vi "Get Slew Rates.vi"(0 "reference in":refnum<class "HPS-17000-PowerModule.lvclass">, 11 "Error In":errorcluster) -> (4 "reference out":refnum<class "HPS-17000-PowerModule.lvclass">, 6 "Slew Rates":T1, 15 "Error Out":errorcluster)   [LabVIEW 2023, in "HPS-17000-PowerModule.lvlib" / "HPS-17000-PowerModule.lvclass"]
uses:
  HPS-17000-PowerModule.lvclass
  builds/PowerModuleInterface/PowerModuleInterface.lvlibp/Classes/PowerModule_interface/Slew Rates.ctl
  HPS-17000-PowerModule.lvclass/HPS-17000-PowerModule.ctl
  builds/PowerModuleInterface/PowerModuleInterface.lvlibp/Classes/PowerModule_interface/PowerModuleInterface.lvclass
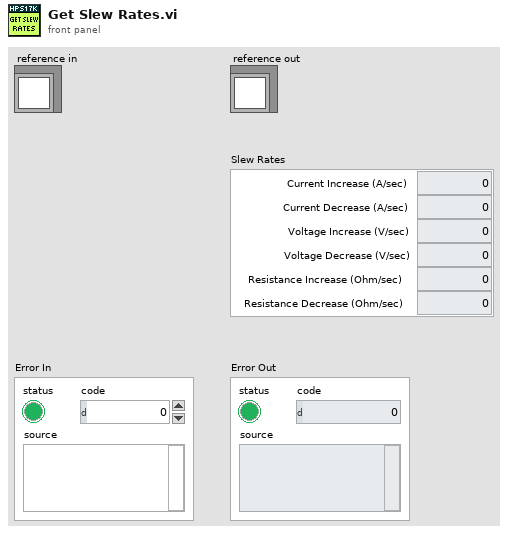
[diagram p1: front panel]
types:
  T1 = typedef "PowerModuleInterface.lvlibp/PowerModuleInterface.lvclass/Slew Rates.ctl" = cluster{"Current Decrease (A/sec)":dbl, "Current Increase (A/sec)":dbl, "Voltage Decrease (V/sec)":dbl, "Voltage Increase (V/sec)":dbl, "Resistance Decrease (Ohm/sec)":dbl, "Resistance Increase (Ohm/sec)":dbl}
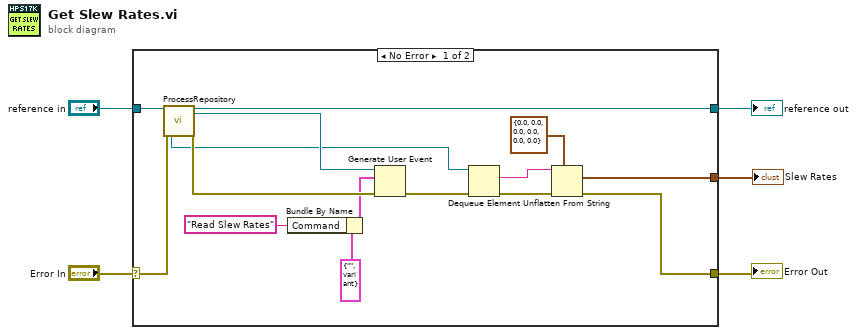
[diagram p0: block diagram]
diagram:
  n1 = case shown="No Error" "Error In" {
    selector: "Error In" -> [w20 w22]
    tunnel: [w9 w22] -> w4
    tunnel: [w18 w21] -> w2
    tunnel: "reference in" -> [w19 w21]
    tunnel: [w6 _] -> w1
    frame No Error {
      n2 = call "ProcessRepository.vi"("reference in"=w19, "Error In"=w20) -> ("QueueFromProcess"=w12:refnum<queue>, "reference out"=w18:refnum<class "HPS-17000-PowerModule.lvclass">, "EventsToProcess"=w17:refnum<user-event>, "Error Out"=w15:errorcluster)  [unwired: 10 in, 4 out]
      n3 = Bundle By Name(cluster=cluster{"Command":string, "Data":variant} {"Command"="", "Data"=variant} ("MessageToProcess"), "Command"="Read Slew Rates") -> (w13:cluster{"Command":string, "Data":variant})
      n4 = Generate User Event(user event=w17, event data cluster=w13, error in=w15) -> (error out=w16:errorcluster)  [unwired: 1 in, 1 out]
      n5 = Dequeue Element(queue=w12, error in (no error)=w16) -> (element=w8:string, error out=w10:errorcluster)  [unwired: 1 in, 2 out]
      n6 = Unflatten From String(type=T1 {"Current Decrease (A/sec)"=0.0, "Current Increase (A/sec)"=0.0, "Voltage Decrease (V/sec)"=0.0, "Voltage Increase (V/sec)"=0.0, "Resistance Decrease (Ohm/sec)"=0.0, "Resistance Increase (Ohm/sec)"=0.0} ("Slew Rates"), binary string=w8, error in (no error)=w10) -> (value=w6:T1, error out=w9:errorcluster)  [unwired: 2 in, 1 out]
    }
    frame Error {
    }
  }
  "Error Out" <- w4
  "reference out" <- w2
  "Slew Rates" <- w1
